vi "render.vi"() -> ()   [LabVIEW 2023]
uses:
  pixel.ctl
panel:
  out "screen":picture
  in  "Pixels":T1[](array[typedef])
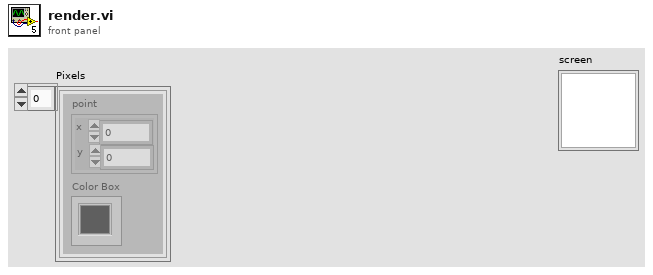
[diagram p1: front panel]
types:
  T1 = typedef "pixel.ctl" = cluster{"point":cluster{"x":i16, "y":i16}, "Color Box":u32}
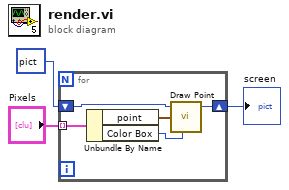
[diagram p0: block diagram]
diagram:
  n1 = for {
    shift-right: [w7] -> w2
    shift-left: picture data[5B] ("screen") -> [w8]
    tunnel: "Pixels" -> [w6] mode=indexing
    n2 = Unbundle By Name(w6) -> ("point"=w5:cluster{"x":i16, "y":i16}, "Color Box"=w4:u32)
    n3 = call <vilib>:"Draw Point.vi"("picture"=w8, "point(x,y)"=w5, "color(black)"=w4) -> ("new picture"=w7:picture)  [unwired: 6 in]
  }
  "screen" <- w2
